vi "Home Move.vi"(7 "Home Pos Shift":dbl, 8 "error in (no error)":errorcluster, 9 "Home Mode":T1=enum."EZ only", 10 "Home Dir (0: -; 1: +)":T2, 11 "CCD in":refnum<class "Motor.lvclass">) -> (0 "error out":errorcluster, 3 "CCD out":refnum<class "Motor.lvclass">)   [LabVIEW 2016, in "Hardware.lvlib" / "Motor.lvlib" / "Motor.lvclass"]
uses:
  <userlib>/Common Components/Hardware/Motor/Motor/Motor.lvclass
  <userlib>/Common Components/Hardware/Motor/Motor/Home Dir.ctl
  <userlib>/Common Components/Hardware/Motor/Motor/Home Mode.ctl
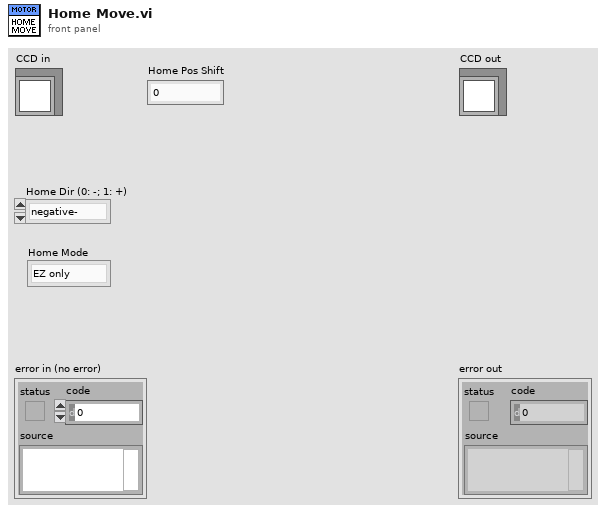
[diagram p1: front panel]
types:
  T1 = typedef "Hardware.lvlib/Motor.lvlib/Motor.lvclass/Home Mode.ctl" = enum16{"EZ+EL", "EZ only"}
  T2 = typedef "Hardware.lvlib/Motor.lvlib/Motor.lvclass/Home Dir.ctl" = enum16{"negative-", "positive+"}
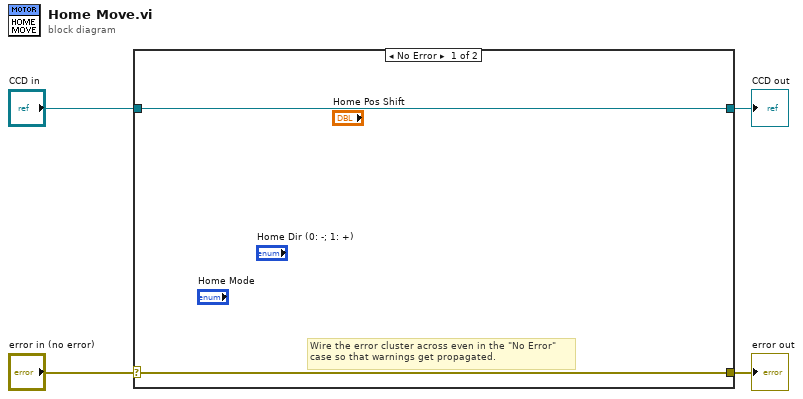
[diagram p0: block diagram]
diagram:
  n1 = case shown="No Error" "error in (no error)" {
    selector: "error in (no error)" -> [w5 w8]
    tunnel: [w5 w8] -> w3
    tunnel: [w6 w7] -> w1
    tunnel: "CCD in" -> [w6 w7]
    frame No Error {
      # "Wire the error cluster across even in the \"No Error\"\ncase so that warnings get propagated."
    }
    frame Error {
    }
  }
  "error out" <- w3
  "CCD out" <- w1
